vi "2 - Temp.vi"() -> ()   [LabVIEW 2023]
panel:
  in  "ON/OFF":bool
  in  "Farenheit":dbl(slide) caption="F" scale=0.0..200.0
  out "Celcius":dbl(slide) scale=0.0..100.0
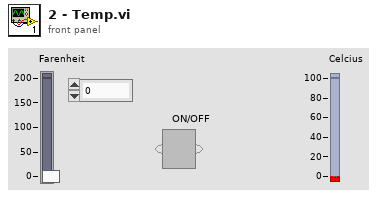
[diagram p1: front panel]
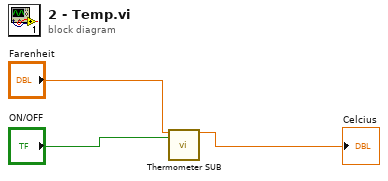
[diagram p0: block diagram]
diagram:
  n1 = call "Thermometer SUB.vi"("Slide"="Farenheit", "Boolean"="ON/OFF") -> ("Numeric"=→"Celcius":dbl)  [unwired: 17 in]
